vi "array_new.vi"(9 "end":dbl=1.0, 10 "size":dbl, 11 "start":dbl) -> (1 "size":i32, 3 "Array":dbl[](array[numeric]))   [LabVIEW 2015]
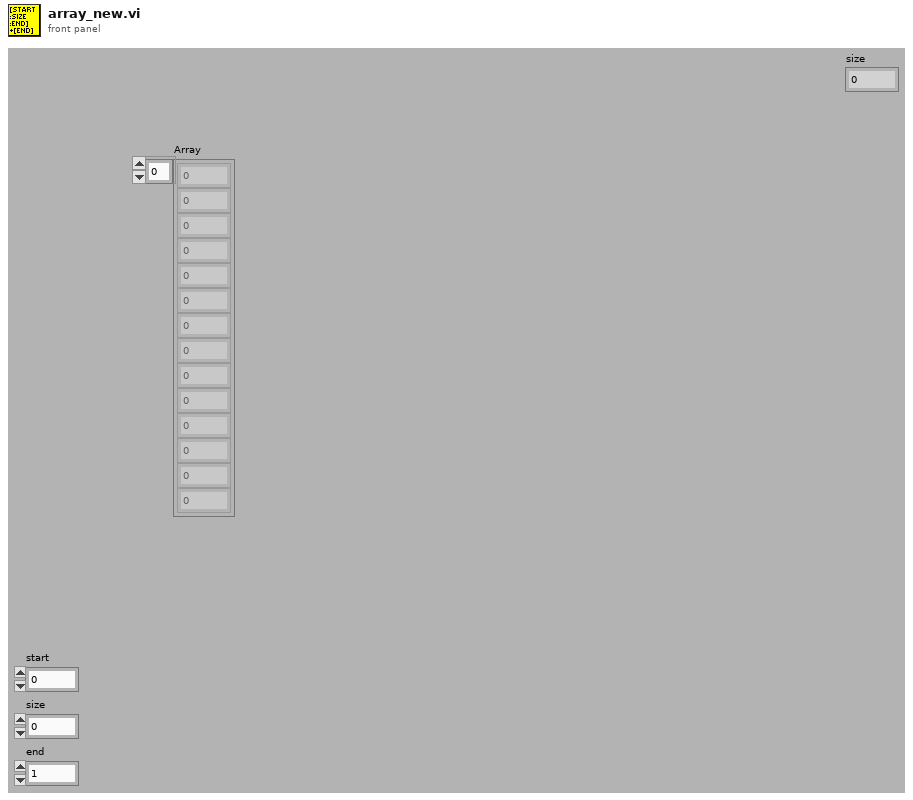
[diagram p1: front panel]
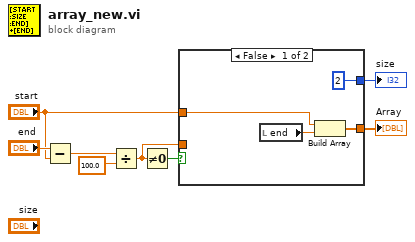
[diagram p0: block diagram]
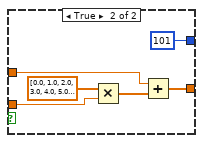
[diagram p2: hidden frame]
diagram:
  n1 = Subtract(x="end", y="start") -> (x-y=w5:dbl)
  n2 = Divide(x=w5, y=100.0) -> (x/y=w3:dbl)
  n3 = Not Equal To 0?(x=w3) -> (x != 0?=w8:bool)
  n4 = case shown="False" w8 {
    tunnel: [w12 w16] -> w7
    tunnel: w3 -> [_ w17]
    tunnel: "start" -> [w10 w15]
    tunnel: [2 101] -> w1
    frame False {
      n5 = local read "end"() -> (w11:dbl)
      n6 = Build Array(w10, w11) -> (w12:dbl[])
    }
    frame True {
      n7 = Multiply(x=dbl[] [0.0, 1.0, 2.0, 3.0, 4.0, 5.0, 6.0, 7.0, 8.0, 9.0, 10.0, 11.0, 12.0, 13.0, 14.0, 15.0, 16.0, 17.0, 18.0, 19.0, 20.0, 21.0, 22.0, 23.0, 24.0, 25.0, 26.0, 27.0, 28.0, 29.0, 30.0, 31.0, 32.0, 33.0, 34.0, 35.0, 36.0, 37.0, 38.0, 39.0, 40.0, 41.0, 42.0, 43.0, 44.0, 45.0, 46.0, 47.0, 48.0, 49.0, 50.0, 51.0, 52.0, 53.0, 54.0, 55.0, 56.0, 57.0, 58.0, 59.0, 60.0, 61.0, 62.0, 63.0, 64.0, 65.0, 66.0, 67.0, 68.0, 69.0, 70.0, 71.0, 72.0, 73.0, 74.0, 75.0, 76.0, 77.0, 78.0, 79.0, 80.0, 81.0, 82.0, 83.0, 84.0, 85.0, 86.0, 87.0, 88.0, 89.0, 90.0, 91.0, 92.0, 93.0, 94.0, 95.0, 96.0, 97.0, 98.0, 99.0, 100.0] ("Array"), y=w17) -> (x*y=w14:dbl[])
      n8 = Add(x=w15, y=w14) -> (x+y=w16:dbl[])
    }
  }
  "Array" <- w7
  "size" <- w1
